vi "ENPH 354 Assignment 1 - Q6.vi"() -> ()   [LabVIEW 2021]
panel:
  out "Negative":dbl[](array[numeric])
  out "Positive":dbl[](array[numeric])
  in  "Array":dbl[](array[numeric])
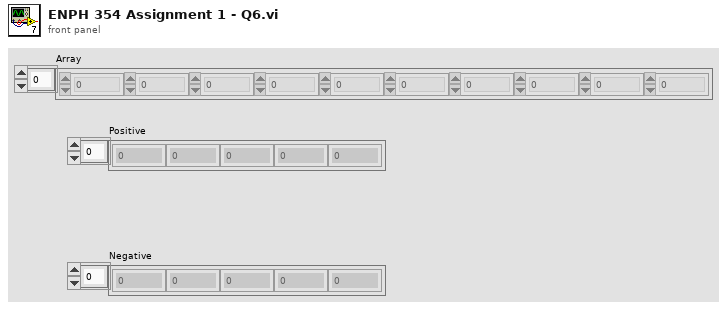
[diagram p1: front panel]
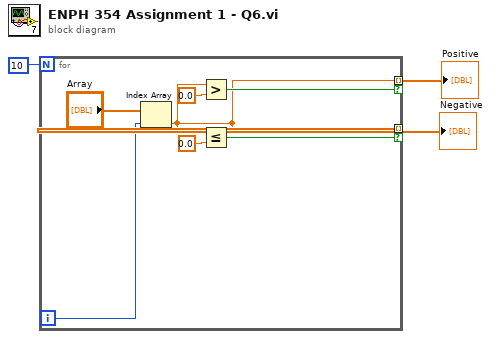
[diagram p0: block diagram]
diagram:
  n1 = for {
    N: 10 -> [_]
    tunnel: [w4] -> w1 mode=indexing if=w5
    tunnel: [w4] -> w2 mode=indexing if=w6
    i -> [w9]
    n2 = Index Array(array="Array", index=w9) -> (element=w4:dbl)
    n3 = Greater?(x=w4, y=0.0) -> (0:w6:bool)
    n4 = Less Or Equal?(x=w4, y=0.0) -> (x <= y?=w5:bool)
  }
  "Negative" <- w1
  "Positive" <- w2
